vi "Message Data Type.vi"(11 "Message Type":string) -> (2 "error out":errorcluster, 3 "Group Data Type":T1)   [LabVIEW 2020, in "Vecto.lvlib" / "RemoteDataService.lvclass"]
uses:
  RemoteDataService.lvclass
  Group Data Type.ctl
  RemoteDataService.lvclass/RemoteDataService.ctl
  VectoConfig/VectoConfig.lvlib
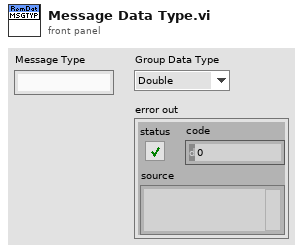
[diagram p1: front panel]
types:
  T1 = typedef "VectoConfig.lvlib/Group Data Type.ctl" = enum16{"Double", "String", "Bool"}
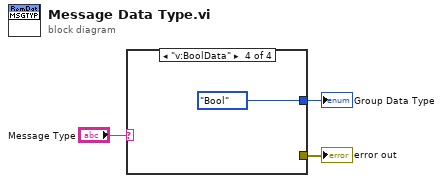
[diagram p0: block diagram]
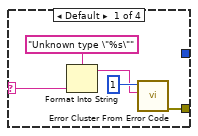
[diagram p2: hidden frame]
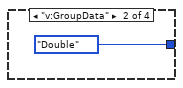
[diagram p3: hidden frame]
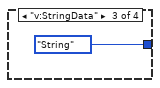
[diagram p4: hidden frame]
diagram:
  n1 = case shown="\"v:BoolData\"" "Message Type" {
    selector: "Message Type" -> [w6 _ _ _]
    tunnel: [_ Group_Data_Type."Double" ("Group Data Type") Group_Data_Type."String" ("Group Data Type") Group_Data_Type."Bool" ("Group Data Type")] -> w2
    tunnel: [w4 _ _ _] -> w1
    frame Default {
      n2 = Format Into String(format string="Unknown type \"%s\"", w6) -> (resulting string=w7:string)  [unwired: 2 in, 1 out]
      n3 = call <vilib>:"Error Cluster From Error Code.vi"("error message (\"\")"=w7, "error code (0)"=1) -> ("error out"=w4:errorcluster)  [unwired: 7 in]
    }
    frame "v:GroupData" {
    }
    frame "v:StringData" {
    }
    frame "v:BoolData" {
    }
  }
  "Group Data Type" <- w2
  "error out" <- w1
